vi "Create DynamicParameter.vi"(5 "AutoKey":string, 7 "RequestedFields":string[](array[string]), 8 "error in (no error)":errorcluster, 9 "ParameterValues":variant[](array[variant]), 10 "ParameterNames":string[](array[string]), 11 "SqlMapper in":refnum<class "SqlMapper.lvclass">) -> (0 "error out":errorcluster, 2 "Parameters":refnum<class "DynamicParameters.lvclass">, 3 "SqlMapper out":refnum<class "SqlMapper.lvclass">, 4 "FieldNames":string[](array[string]), 6 "ParameterNames":string[](array[string]))   [LabVIEW 2020, in "ORM.lvlib" / "TypeMap.lvclass"]
uses:
  TypeMap.lvclass
  DynamicParameters/DynamicParameters.lvclass
  SqlMapper/SqlMapper.lvclass
  SqlMapper/SqlMapper.lvclass/SqlMapper.ctl
  DynamicParameters/DynamicParameters.lvclass/DynamicParameters.ctl
  SqlMapper/Read DbConnection.vi
  SqlMapper/Write DbConnection.vi
  DynamicParameters/Write FieldNames.vi
  DynamicParameters/Write AutoKey.vi
  DynamicParameters/Write RequestedFields.vi
  DbConnection/DbConnection.lvclass
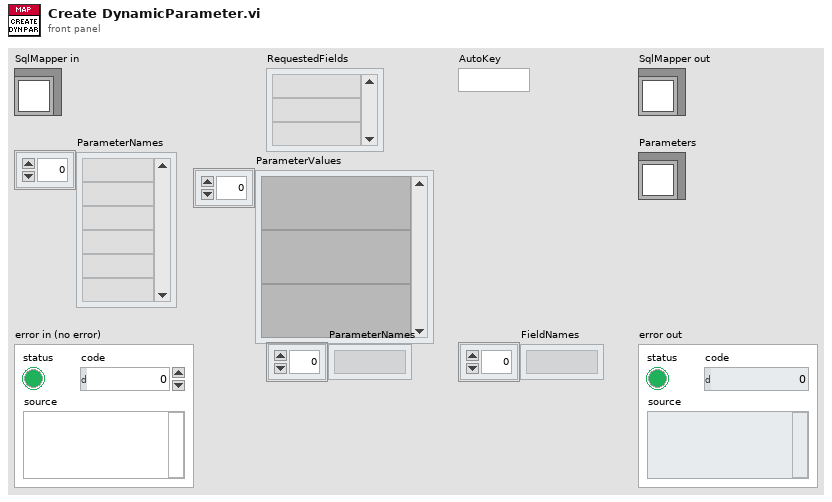
[diagram p1: front panel]
types:
  T1 = cluster{"DbType":i32, "Direction":i32, "Size":i32, "Precision":u8, "Scale":u8}
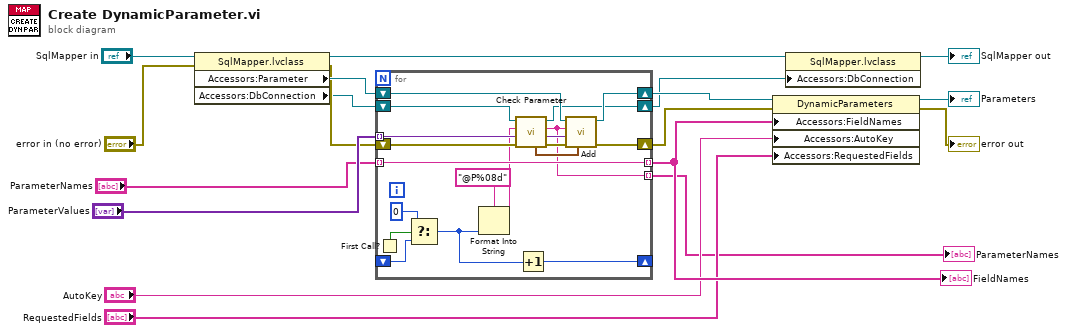
[diagram p0: block diagram]
diagram:
  n1 = property class="SqlMapper.lvclass"(reference="SqlMapper in", error in="error in (no error)") -> (reference out=w11:refnum<class "SqlMapper.lvclass">, error out=w7:errorcluster, "Accessors:Parameter"=w12:refnum<class "DynamicParameters.lvclass">, "Accessors:DbConnection"=w4:refnum<class "DbConnection.lvclass">)
  n2 = for {
    shift-right: [w37] -> w9
    shift-left: w12 -> [w36]
    tunnel: "ParameterNames" -> [w33] mode=indexing
    tunnel: "ParameterValues" -> [w32] mode=indexing
    shift-right: [w35] -> w17
    shift-left: w7 -> [w31]
    tunnel: [w24] -> w3 mode=indexing
    tunnel: [w33] -> w14 mode=indexing
    shift-right: [w25] -> w1
    shift-left: w4 -> [w26]
    shift-right: [w23] -> _
    shift-left: _ -> [w21]
    n3 = First Call?() -> (First Call?: T/F=w19:bool)
    n4 = Select(t=0, s=w19, f=w21) -> (s? t:f=w20:i32)
    n5 = Format Into String(format string="@P%08d", w20) -> (resulting string=w27:string)  [unwired: 2 in, 1 out]
    n6 = call-dynamic "Check Parameter.vi"("error in (no error)"=w31, "value in"=w32, "name in"=w27, "DbConnection in"=w26) -> ("error out"=w30:errorcluster, "value out"=w28:variant, "name out"=w24:string, "DbConnection out"=w25:refnum<class "DbConnection.lvclass">, "Options out"=w29:T1)  [unwired: 3 in]
    n7 = Increment(x=w20) -> (x+1=w23:i32)
    n8 = call-dynamic "Add.vi"("Options"=w29, "error in (no error)"=w30, "value"=w28, "name"=w24, "DynamicParameters in"=w36) -> ("error out"=w35:errorcluster, "DynamicParameters out"=w37:refnum<class "DynamicParameters.lvclass">)  [unwired: 5 in]
  }
  "FieldNames" <- w14
  "ParameterNames" <- w3
  n9 = property class="DynamicParameters"(reference=w9, error in=w17, "Accessors:FieldNames"=w14, "Accessors:AutoKey"="AutoKey", "Accessors:RequestedFields"="RequestedFields") -> (reference out=→"Parameters":refnum<class "DynamicParameters.lvclass">, error out=→"error out":errorcluster)
  n10 = property class="SqlMapper.lvclass"(reference=w11, "Accessors:DbConnection"=w1) -> (reference out=→"SqlMapper out":refnum<class "SqlMapper.lvclass">)  [unwired: 1 in, 1 out]
